vi "TrajectoryCalculateOrientationTowards.vi"(5 "Starting Fraction":dbl=0.25, 6 "Init":bool, 7 "Completion Fraction":dbl=0.75, 8 "Total Trajectory Time Sec":dbl, 9 "Elapsed Traj Time Sec":dbl, 10 "Current Orientation Demand DEG":dbl, 11 "Starting Orientation  DEG":dbl) -> (1 "Rotational Velocity Rad Per Sec":dbl, 2 "Orientation Demand Deg":dbl, 3 "Orientation Demand":T1 {"SIN" format="%13.4f"; "COS" format="%13.4f"; "VALUE" format="%13.4f"})   [LabVIEW 2023]
uses:
  <vilib>/Rock Robotics/WPI/ThirdParty/JAS_Junk/TrajLib/TypeDef/ROTATION2D.ctl
  <vilib>/Rock Robotics/WPI/ThirdParty/JAS_Junk/TrajLib/Rotation2d_CreateAngle.vi
  <vilib>/Rock Robotics/WPI/ThirdParty/JAS_Junk/TrajLib/Rotation2d_Plus.vi
  <vilib>/Rock Robotics/WPI/ThirdParty/JAS_Junk/TrajLib/Rotation2d_Times.vi
  <vilib>/Rock Robotics/WPI/ThirdParty/JAS_Junk/TrajLib/Rotation2d_UnaryMinus.vi
  <vilib>/Rock Robotics/WPI/ThirdParty/JAS_Junk/TrajLib/Rotation2d_RotateBy.vi
  <vilib>/Rock Robotics/WPI/ThirdParty/JAS_Junk/TrajLib/Rotation2d_GetRadians.vi
  <vilib>/Rock Robotics/WPI/ThirdParty/JAS_Junk/TrajLib/Conv_Radians_Deg.vi
  <vilib>/Rock Robotics/WPI/ThirdParty/JAS_Junk/TrajLib/Rotation2d_CreateXY.vi
  <vilib>/Rock Robotics/WPI/ThirdParty/JAS_Junk/TrajLib/Util_CalcDist.vi
  <vilib>/Rock Robotics/WPI/ThirdParty/JAS_Junk/TrajLib/Trajectory_Library.lvlib
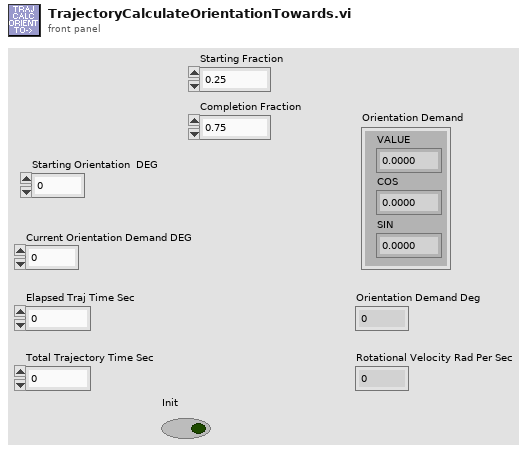
[diagram p1: front panel]
types:
  T1 = typedef "Trajectory_Library.lvlib/ROTATION2D.ctl" = cluster{"VALUE":dbl, "COS":dbl, "SIN":dbl}
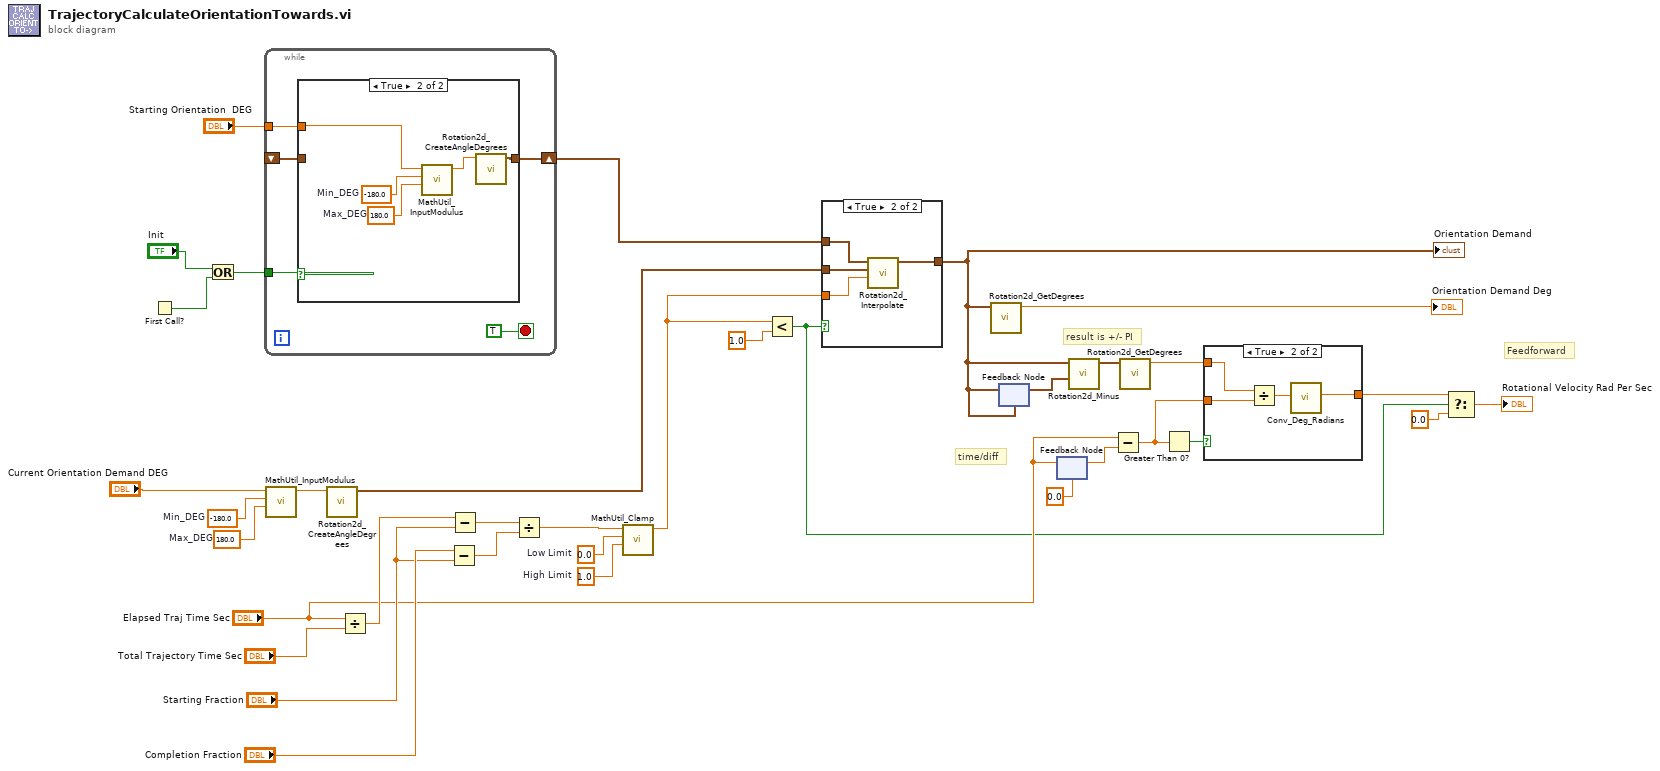
[diagram p0: block diagram]
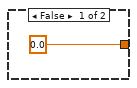
[diagram p2: hidden frame]
diagram:
  w4 = -180.0  # Min_DEG
  w3 = 180.0  # Max_DEG
  w28 = 1.0  # High Limit
  w27 = 0.0  # Low Limit
  # "result is +/- PI"
  # "time/diff"
  # "Feedforward"
  n1 = First Call?() -> (First Call?: T/F=w7:bool)
  n2 = Or(x="Init", y=w7) -> (x .or. y?=w5:bool)
  n3 = while {
    shift-right: [w39] -> w34
    shift-left: _ -> [w38]
    tunnel: "Starting Orientation  DEG" -> [w37]
    tunnel: w5 -> [w36]
    stop <- TRUE stop-if-true
    n4 = case shown="True" w36 {
      tunnel: [w41 w46] -> w39
      tunnel: w38 -> [w41 _]
      tunnel: w37 -> [_ w42]
      frame False {
      }
      frame True {
        w44 = -180.0  # Min_DEG
        w45 = 180.0  # Max_DEG
        n5 = call <vilib>:"MathUtil_InputModulus.vi"("Maximum_Input"=w45, "Minimum_Input"=w44, "Input"=w42) -> ("modulus"=w43:dbl)  [unwired: 8 in]
        n6 = call <vilib>:"Rotation2d_CreateAngleDegrees.vi"("Angle_Degrees"=w43) -> ("ROTATION"=w46:T1)  [unwired: 10 in]
      }
    }
  }
  n7 = call <vilib>:"MathUtil_InputModulus.vi"("Maximum_Input"=w3, "Minimum_Input"=w4, "Input"="Current Orientation Demand DEG") -> ("modulus"=w2:dbl)  [unwired: 8 in]
  n8 = call <vilib>:"Rotation2d_CreateAngleDegrees.vi"("Angle_Degrees"=w2) -> ("ROTATION"=w24:T1)  [unwired: 10 in]
  n9 = Divide(x="Elapsed Traj Time Sec", y="Total Trajectory Time Sec") -> (x/y=w31:dbl)
  n10 = Subtract(x="Completion Fraction", y="Starting Fraction") -> (x-y=w25:dbl)
  n11 = Subtract(x=w31, y="Starting Fraction") -> (x-y=w32:dbl)
  n12 = Divide(x=w32, y=w25) -> (x/y=w26:dbl)
  n13 = call <vilib>:"MathUtil_Clamp.vi"("High Limit"=w28, "Low Limit"=w27, "Value"=w26) -> ("Result"=w23:dbl)  [unwired: 8 in]
  n14 = Less?(x=w23, y=1.0) -> (x < y?=w14:bool)
  n15 = case shown="True" w14 {
    tunnel: w34 -> [_ w51]
    tunnel: w24 -> [w47 w50]
    tunnel: w23 -> [_ w49]
    tunnel: [w47 w48] -> w11
    frame False {
    }
    frame True {
      n16 = call <vilib>:"Rotation2d_Interpolate.vi"("T"=w49, "EncValue ROTATION"=w50, "in ROTATION"=w51) -> ("Interpolated ROTATION"=w48:T1)  [unwired: 8 in]
    }
  }
  "Orientation Demand" <- w11
  n17 = call <vilib>:"Rotation2d_GetDegrees.vi"("in ROTATION"=w11) -> ("AngleDegrees"=→"Orientation Demand Deg":dbl)  [unwired: 10 in]
  n18 = feedback-in #1(w11) -> ()
  n19 = feedback #1(w11) -> (w10:T1)
  n20 = feedback #2(0.0 ("Elapsed Traj Time Sec")) -> (w18:dbl)
  n21 = feedback-in #2("Elapsed Traj Time Sec") -> ()
  n22 = call <vilib>:"Rotation2d_Minus.vi"("other ROTATION"=w10, "in ROTATION"=w11) -> ("out ROTATION"=w9:T1)  [unwired: 9 in]
  n23 = Subtract(x="Elapsed Traj Time Sec", y=w18) -> (x-y=w16:dbl)
  n24 = call <vilib>:"Rotation2d_GetDegrees.vi"("in ROTATION"=w9) -> ("AngleDegrees"=w8:dbl)  [unwired: 10 in]
  n25 = Greater Than 0?(x=w16) -> (x > 0?=w17:bool)
  n26 = case shown="True" w17 {
    tunnel: w16 -> [_ w56]
    tunnel: [0.0 ("Radians") w54] -> w15
    tunnel: w8 -> [_ w53]
    frame False {
    }
    frame True {
      n27 = Divide(x=w53, y=w56) -> (x/y=w55:dbl)
      n28 = call <vilib>:"Conv_Deg_Radians.vi"("Degress"=w55) -> ("Radians"=w54:dbl)  [unwired: 10 in]
    }
  }
  n29 = Select(t=w15, s=w14, f=0.0) -> (s? t:f=→"Rotational Velocity Rad Per Sec":dbl)
